vi "Create build_vip.bat.vi"(7 "template folder":path, 8 "error in (no error)":errorcluster, 10 "VIPB File":path) -> (0 "error out":errorcluster, 2 "build_vip.bat Preview":string, 3 "build_vip.bat path":path)   [LabVIEW 2019, in "VIPM.lvlib"]
uses:
  VIPM.lvlib
  <vilib>/JKI/VIPM API/command-line/support/VI Package Build Spec Data Cluster_vipm_api.ctl
  <vilib>/JKI/VIPM API/command-line/support/Version Info Cluster_vipm_api.ctl
  <vilib>/JKI/VIPM API/VIPM API_vipm_api.lvlib
panel:
  out "Build Spec":T1
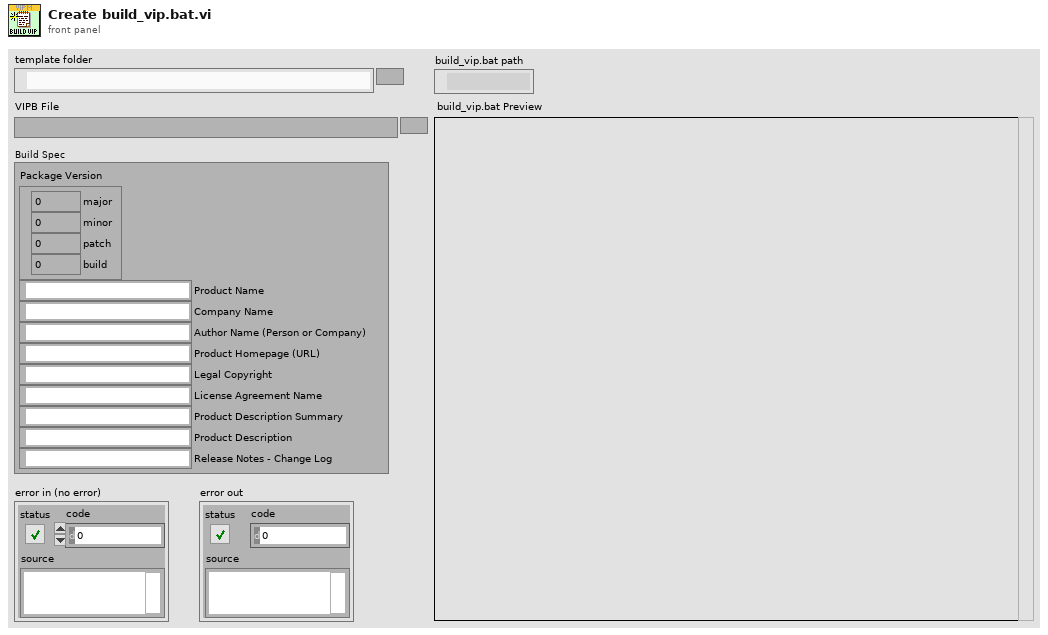
[diagram p1: front panel]
types:
  T1 = typedef "VIPM API_vipm_api.lvlib/VI Package Build Spec Data Cluster_vipm_api.ctl" = cluster{"Package Version":T2, "Product Name":string, "Company Name":string, "Author Name (Person or Company)":string, "Product Homepage (URL)":string, "Legal Copyright":string, "License Agreement Name":string, "Product Description Summary":string, "Product Description":string, "Release Notes - Change Log":string}
  T2 = typedef "VIPM API_vipm_api.lvlib/Version Info Cluster_vipm_api.ctl" = cluster{"major":u32, "minor":u32, "patch":u32, "build":u32}
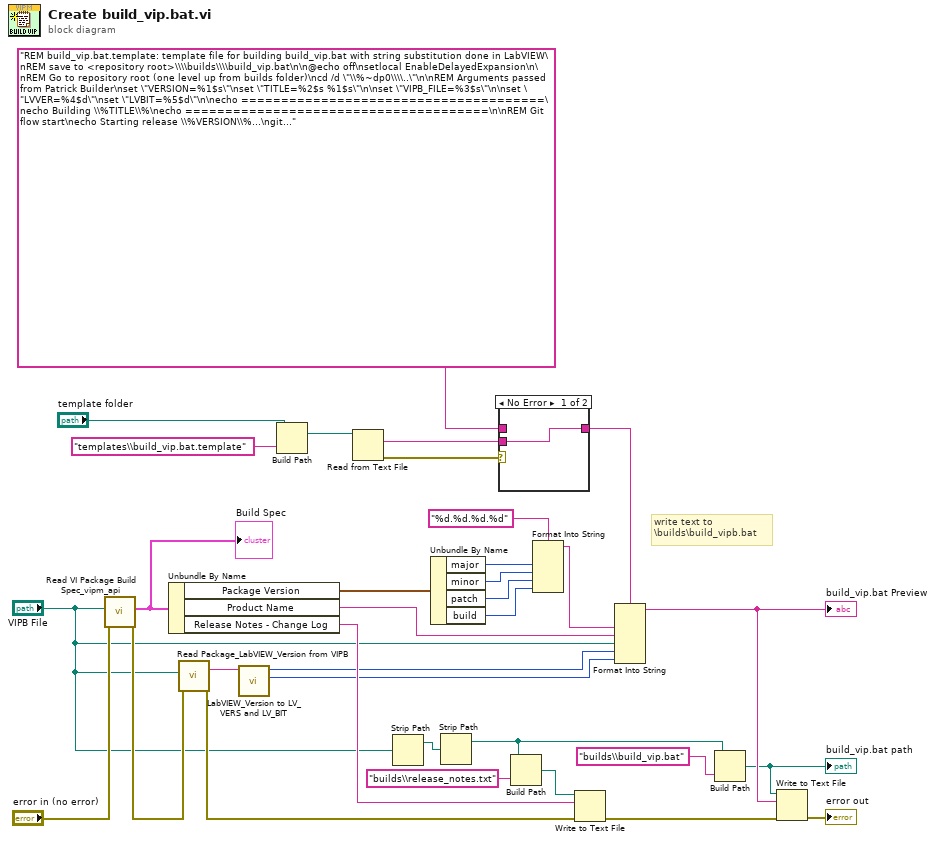
[diagram p0: block diagram]
diagram:
  # "write text to\n\\builds\\build_vipb.bat"
  n1 = call <vilib>:"Read VI Package Build Spec_vipm_api.vi"("error in (no error)"="error in (no error)", "Path to VIPB File"="VIPB File") -> ("error out"=w8:errorcluster, "VI Package Build Spec Data"=w16:T1)  [unwired: 8 in]
  "Build Spec" <- w16
  n2 = Unbundle By Name(w16) -> ("Package Version"=w33:T2, "Product Name"=w32:string, "Release Notes - Change Log"=w24:string)
  n3 = call "Read Package_LabVIEW_Version from VIPB.vi"("error in"=w8, "VIPB File Path"="VIPB File") -> ("error out"=w7:errorcluster, "Package_LabVIEW_Version"=w6:string)  [unwired: 8 in]
  n4 = call "LabVIEW_Version to LV_VERS and LV_BIT.vi"("Package_LabVIEW_Version"=w6) -> ("LV_BIT"=w4:u32, "LV_VER"=w5:u32)  [unwired: 9 in]
  n5 = Build Path(base path="template folder", name or relative path="templates\\build_vip.bat.template") -> (appended path=w12:path)
  n6 = Read from Text File(file (use dialog)=w12) -> (text=w9:string, error out=w11:errorcluster)  [unwired: 3 in, 2 out]
  n7 = Strip Path(path="VIPB File") -> (stripped path=w21:path)  [unwired: 1 out]
  n8 = Unbundle By Name(w33) -> ("major"=w26:u32, "minor"=w30:u32, "patch"=w29:u32, "build"=w28:u32)
  n9 = Strip Path(path=w21) -> (stripped path=w18:path)  [unwired: 1 out]
  n10 = case shown="No Error" w11 {
    tunnel: [w34 w35] -> w10
    tunnel: "REM build_vip.bat.template: template file for building build_vip.bat with string substitution done in LabVIEW\nREM save to <repository root>\\\\builds\\\\build_vip.bat\n\n@echo off\nsetlocal EnableDelayedExpansion\n\nREM Go to repository root (one level up from builds folder)\ncd /d \"\\%~dp0\\\\..\"\n\nREM Arguments passed from Patrick Builder\nset \"VERSION=%1$s\"\nset \"TITLE=%2$s %1$s\"\n\nset \"VIPB_FILE=%3$s\"\n\nset \"LVVER=%4$d\"\nset \"LVBIT=%5$d\"\n\necho ======================================\necho Building \\%TITLE\\%\necho ======================================\n\nREM Git flow start\necho Starting release \\%VERSION\\%...\ngit flow release start \\%VERSION\\%\nif \\%ERRORLEVEL\\% neq 0 (\n    echo ERROR: git flow release start failed\n    goto error_handler\n)\n\nREM Archive old releases\necho Archiving previous release...\nif not exist \"builds\\\\old releases\" mkdir \"builds\\\\old releases\"\n\nif exist \"builds\\\\latest\\\\*.*\" (\n    move /Y \"builds\\\\latest\\\\*.*\" \"builds\\\\old releases\\\\\"\n) else (\n    if not exist \"builds\\\\latest\" mkdir \"builds\\\\latest\"\n)\n\nREM Build VIP\necho Building VIP...\ng-cli --lv-ver \\%LVVER\\% --arch \\%LVBIT\\% vipBuild -- \"\\%VIPB_FILE\\%\"\nif \\%ERRORLEVEL\\% neq 0 (\n    echo ERROR: VIP build failed\n    goto error_handler\n)\n\nREM Execute generated script (builds exe/installer/7z) - if it exists\nif exist \"builds\\\\7z Install\\\\7zip.bat\" (\n    echo Building executables and installers...\n    call \"builds\\\\7z Install\\\\7zip.bat\"\n    if \\%ERRORLEVEL\\% neq 0 (\n        echo ERROR: Executable build failed\n        goto error_handler\n    )\n) else (\n    echo Skipping executable/installer build ^(7zip.bat not found^)\n)\n\nREM Git flow finish\necho Committing changes...\ngit commit -m \"Build \\%VERSION\\%\" -a\nif \\%ERRORLEVEL\\% neq 0 (\n    echo ERROR: git commit failed\n    goto error_handler\n)\n\necho Finishing release \\%VERSION\\%...\ngit flow release finish \\%VERSION\\% -m \"Build \\%VERSION\\%\"\nif \\%ERRORLEVEL\\% neq 0 (\n    echo ERROR: git flow release finish failed\n    goto error_handler\n)\n\ngit reset --hard\nif \\%ERRORLEVEL\\% neq 0 (\n    echo ERROR: git reset failed\n    exit /b 1\n)\n\necho Pushing to remote...\ngit push --all\nif \\%ERRORLEVEL\\% neq 0 (\n    echo ERROR: git push --all failed\n    exit /b 1\n)\n\ngit push --tags\nif \\%ERRORLEVEL\\% neq 0 (\n    echo ERROR: git push --tags failed\n    exit /b 1\n)\n\nREM GitHub release\necho Creating GitHub release \\%VERSION\\%...\n\nREM Notes written to builds\\release_notes.txt by Patrick Builder\n\nset ASSETS=\nfor \\%\\%F in (builds\\\\latest\\\\*.vip builds\\\\latest\\\\*.exe) do (\n    set ASSETS=!ASSETS! \"\\%\\%F\"\n)\ngh release create \\%VERSION\\% !ASSETS! -t \"\\%TITLE\\%\" -F builds\\\\release_notes.txt\nif \\%ERRORLEVEL\\% neq 0 (\n    echo ERROR: GitHub release creation failed\n    exit /b 1\n)\n\nREM Clean up temp file\ndel builds\\\\release_notes.txt\n\necho.\necho ======================================\necho Build \\%VERSION\\% completed successfully\necho ======================================\nexit /b 0\n\n:error_handler\necho.\necho ==========================================\necho BUILD FAILED - Cleaning up git state\necho ==========================================\n\nREM Try git flow delete first\ngit flow release delete \\%VERSION\\% 2>nul\n\nREM If that didn't work, manual cleanup\ngit checkout develop 2>nul\ngit branch -D release\\%VERSION\\% 2>nul\n\nexit /b 1" ("format string") -> [_ w35]
    tunnel: w9 -> [w34 _]
    frame No Error {
    }
    frame Error {
    }
  }
  n11 = Build Path(base path=w18, name or relative path="builds\\release_notes.txt") -> (appended path=w23:path)
  n12 = Format Into String(format string="%d.%d.%d.%d", w26, w30, w29, w28) -> (resulting string=w27:string)  [unwired: 2 in, 1 out]
  n13 = Write to Text File(file (use dialog)=w23, text=w24, error in=w7) -> (error out=w20:errorcluster)  [unwired: 1 in, 2 out]
  n14 = Format Into String(format string=w10, w27, w32, "VIPB File", w5, w4) -> (resulting string=w17:string)  [unwired: 2 in, 1 out]
  "build_vip.bat Preview" <- w17
  n15 = Build Path(base path=w18, name or relative path="builds\\build_vip.bat") -> (appended path=w15:path)
  "build_vip.bat path" <- w15
  n16 = Write to Text File(file (use dialog)=w15, text=w17, error in=w20) -> (error out=→"error out":errorcluster)  [unwired: 1 in, 2 out]
